vi "Get Contents.vi"(8 "error in (no error)":errorcluster, 11 "List in":refnum<class "List.lvclass">) -> (0 "error out":errorcluster, 2 "Contents":string[][](array[string]), 3 "List out":refnum<class "List.lvclass">)   [LabVIEW 2015, in "List.lvclass"]
uses:
  List.lvclass
  List.lvclass/List.ctl
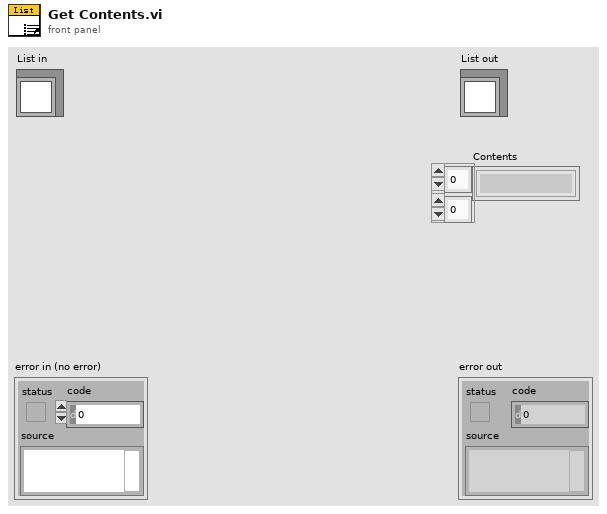
[diagram p1: front panel]
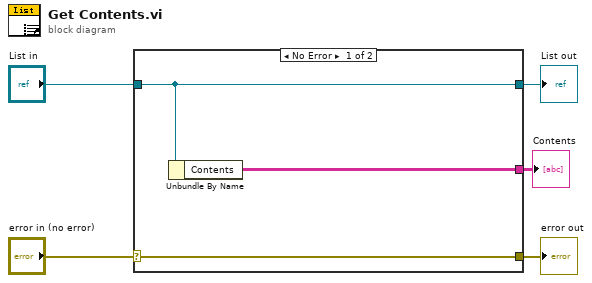
[diagram p0: block diagram]
diagram:
  n1 = case shown="No Error" "error in (no error)" {
    selector: "error in (no error)" -> [w8 w9]
    tunnel: [w8 w9] -> w4
    tunnel: [w7 w10] -> w2
    tunnel: "List in" -> [w7 w10]
    tunnel: [w6 _] -> w1
    frame No Error {
      n2 = Unbundle By Name(w7) -> ("Contents"=w6:string[][])
    }
    frame Error {
    }
  }
  "error out" <- w4
  "List out" <- w2
  "Contents" <- w1
